vi "Teleop_debugging.vi"(10 "Match Info":T1={"Autonomous Elapsed Seconds"=0.0, "TeleOp Elapsed Seconds"=0.0, "Disabled Elapsed Seconds"=0.0, "Visited Autonomous"=FALSE, "Visited TeleOp"=FALSE, "Visited Disabled"=FALSE, "Autonomous Settings"={"Autonomous Style"=enum."Independent", "VI Refnum"=refnum}}, 11 "Call Context":T2) -> ()   [LabVIEW 2011]
doc: "This VI is called for each TeleOp packet received from the DS where the robot is not disabled. It is often used to read from the joysticks and update I/O or to update setpoints for timed control loops. It should complete and return within 20 milliseconds or it may miss DS packets."
uses:
  <vilib>/Rock Robotics/WPI/DriverStation/WPI_DriverStationDerivedRobotMode.ctl
  <vilib>/Rock Robotics/WPI/DriverStation/WPI_DriverStationMatch Info.ctl
  <vilib>/Rock Robotics/WPI/DriverStation/DriverStationLCD/WPI_DriverStationLCDLCDLine.ctl
  Robot Global Data.vi
  <vilib>/Rock Robotics/WPI/RobotDrive/WPI_RobotDriveMecanumDrive_Cartesian.vi
  <vilib>/addons/control/pid/NI_PID_pid.lvlib
panel:
  in  "ShooterAngle3":cluster{"time":dbl, "Arm Pos 1":dbl}[](array[cluster])=[{"time"=2.2540983606557377, "Arm Pos 1"=-0.5639931736228638}] {"Arm Pos 1" scale=1.0..-1.0 scale format="%#_4g"; "time" scale=0.0..5.0}
  in  "ShooterAngle2":cluster{"time":dbl, "Arm Pos 1":dbl}[](array[cluster])=[{"time"=2.2540983606557377, "Arm Pos 1"=-0.5639931736228638}] {"Arm Pos 1" scale=1.0..-1.0 scale format="%#_4g"; "time" scale=0.0..5.0}
  in  "ShooterAngle1":cluster{"time":dbl, "Arm Pos 1":dbl}[](array[cluster])=[{"time"=2.2540983606557377, "Arm Pos 1"=-0.5639931736228638}] {"Arm Pos 1" scale=1.0..-1.0 scale format="%#_4g"; "time" scale=0.0..5.0}
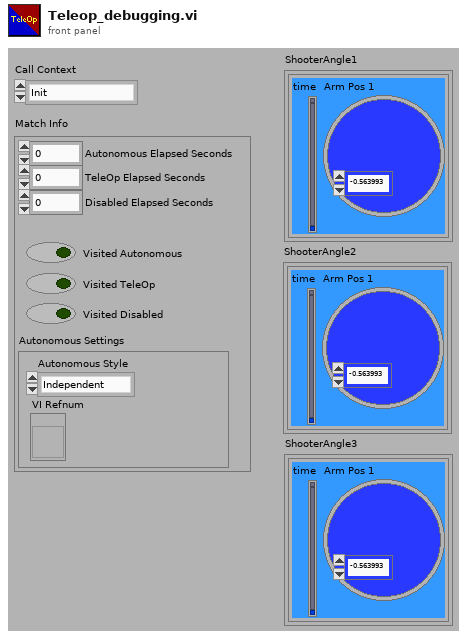
[diagram p1: front panel]
types:
  T1 = typedef "WPI_DriverStationMatch Info.ctl" = cluster{"Autonomous Elapsed Seconds":dbl, "TeleOp Elapsed Seconds":dbl, "Disabled Elapsed Seconds":dbl, "Visited Autonomous":bool, "Visited TeleOp":bool, "Visited Disabled":bool, "Autonomous Settings":cluster{"Autonomous Style":enum16{"Iterative", "Independent"}, "VI Refnum":refnum<vi>}}
  T2 = typedef "WPI_DriverStationDerivedRobotMode.ctl" = enum16{"Init", "Execute", "Stop"}
  T3 = typedef "WPI_DriverStationLCDLCDLine.ctl" = enum16{"Main - Line 1", "User - Line 2", "User - Line 3", "User - Line 4", "User - Line 5", "User - Line 6"}
  T4 = typedef "WPI_JoystickDevRef.ctl" = cluster{"Device":T5}
  T5 = typedef "WPI_JoystickDeviceEnum.ctl" = enum16{"USB 1", "USB 2", "USB 3", "USB 4", "Kinect 1", "Kinect 2"}
  T6 = typedef "WPI_MotorControlDeviceRef.ctl" = cluster{"DeviceStatus":errorcluster, "Type":enum16{"PWM", "CAN"}, "PWM":cluster{"Digital Module":T7, "PWM Channel":T8, "DeadBand":T9}, "CAN":cluster{"Device Number":u8, "Control Mode":T10, "Semaphore":T11, "Max Vout":dbl}, "Invert":bool, "TransformRef":T12, "InvTransformRef":T12}
  T7 = typedef "FPGA_TypedefDigitalModule.ctl" = enum16{"Digital Module 1", "Digital Module 2"}
  T8 = typedef "FPGA_DIOPWMChannel.ctl" = enum8{"PWM 1", "PWM 2", "PWM 3", "PWM 4", "PWM 5", "PWM 6", "PWM 7", "PWM 8", "PWM 9", "PWM 10", "Invalid"}
  T9 = typedef "WPI_PWMDeadband.ctl" = cluster{"Name":string, "maxPositivePwm":i32, "minPositivePwm":i32, "centerPwm":i32, "maxNegativePwm":i32, "minNegativePwm":i32, "angularRange":u16}
  T10 = typedef "WPI_CANJaguar_ControlMode.ctl" = enum8{"Percent VBus", "Current", "Speed", "Position", "Voltage"}
  T11 = typedef "Semaphore RefNum" = refnum<k1>
  T12 = typedef "WPI_PWMTransform_ConPane.ctl" = refnum<vi>
  T13 = cluster{"axis 1 (x)":dbl, "axis 2 (y)":dbl, "axis 3 (throttle)":dbl, "axis 4":dbl, "axis 5":dbl, "axis 6":dbl}
  T14 = typedef "WPI_JoystickButtonState.ctl" = cluster{"Button 1":bool, "Button 2":bool, "Button 3":bool, "Button 4":bool, "Button 5":bool, "Button 6":bool, "Button 7":bool, "Button 8":bool, "Button 9":bool, "Button 10":bool, "Button 11":bool, "Button 12":bool}
  T15 = typedef "WPI_ServoDeviceRef.ctl" = cluster{"DeviceStatus":errorcluster, "Digital Module":T7, "PWM Channel":T8, "DeadBand":T9}
  T16 = typedef "WPI_RobotDriveDevRef.ctl" = cluster{"DevStatus":errorcluster, "Motors[]":T6[], "Square Inputs":bool, "Max Output":dbl, "Isochronous":bool}
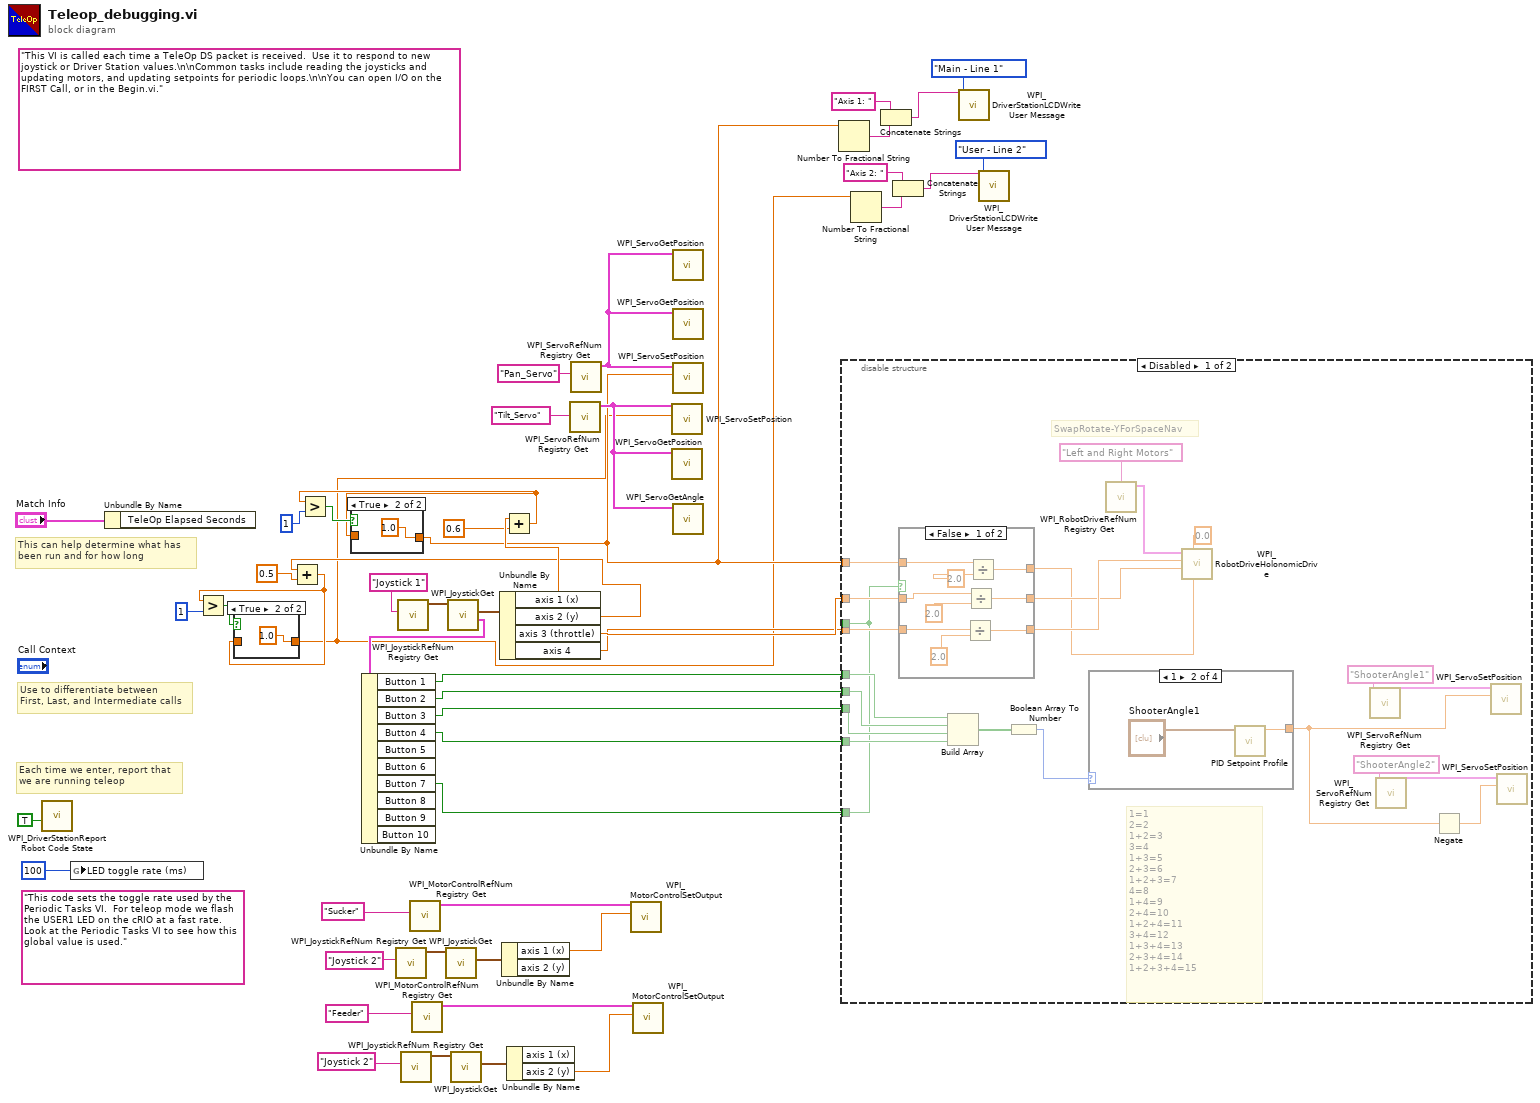
[diagram p0: block diagram]
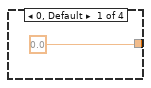
[diagram p4: hidden frame]
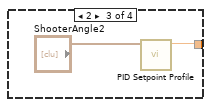
[diagram p5: hidden frame]
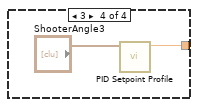
[diagram p6: hidden frame]
diagram:
  (unwired) "This code sets the toggle rate used by the Periodic Tasks VI.  For teleop mode we flash the USER1 LED on the cRIO at a fast rate.  Look at the Periodic Tasks VI to see how this global value is used."
  (unwired) "This VI is called each time a TeleOp DS packet is received.  Use it to respond to new joystick or Driver Station values.\n\nCommon tasks include reading the joysticks and updating motors, and updating setpoints for periodic loops.\n\nYou can open I/O on the FIRST Call, or in the Begin.vi."
  # "Each time we enter, report that\nwe are running teleop"
  # "Use to differentiate between\nFirst, Last, and Intermediate calls"
  # "This can help determine what has\nbeen run and for how long"
  n1 = call <vilib>:"WPI_DriverStationReport Robot Code State.vi"("TeleOp"=TRUE ("Autonomous")) -> ()  [unwired: 10 in, 1 out]
  n2 = global write "Robot Global Data.vi" "LED toggle rate (ms)"(u32 100 ("LED ms toggle rate")) -> ()
  n3 = Unbundle By Name("Match Info") -> ()  [unwired: 1 out]
  n4 = call <vilib>:"WPI_JoystickRefNum Registry Get.vi"("refnum name"="Joystick 2") -> ("JoystickDevRef"=w45:T4)  [unwired: 1 in, 9 out]
  n5 = call <vilib>:"WPI_JoystickRefNum Registry Get.vi"("refnum name"="Joystick 1") -> ("JoystickDevRef"=w33:T4)  [unwired: 1 in, 9 out]
  n6 = call <vilib>:"WPI_JoystickRefNum Registry Get.vi"("refnum name"="Joystick 2") -> ("JoystickDevRef"=w39:T4)  [unwired: 1 in, 9 out]
  n7 = call <vilib>:"WPI_MotorControlRefNum Registry Get.vi"("refnum name"="Sucker") -> ("MotorControlDevRef"=w44:T6)  [unwired: 9 in, 1 out]
  n8 = call <vilib>:"WPI_MotorControlRefNum Registry Get.vi"("refnum name"="Feeder") -> ("MotorControlDevRef"=w38:T6)  [unwired: 9 in, 1 out]
  n9 = call <vilib>:"WPI_JoystickGet.vi"("JoystickDevRef"=w45) -> ("Axes"=w47:T13)  [unwired: 1 in, 5 out]
  n10 = call <vilib>:"WPI_JoystickGet.vi"("JoystickDevRef"=w33) -> ("Buttons"=w32:T14, "Axes"=w35:T13)  [unwired: 1 in, 4 out]
  n11 = Unbundle By Name(w32) -> ("Button 1"=w29:bool, "Button 2"=w28:bool, "Button 3"=w27:bool, "Button 4"=w26:bool, "Button 7"=w25:bool)  [unwired: 5 out]
  n12 = call <vilib>:"WPI_JoystickGet.vi"("JoystickDevRef"=w39) -> ("Axes"=w41:T13)  [unwired: 1 in, 5 out]
  n13 = Unbundle By Name(w35) -> ("axis 1 (x)"=w12:dbl, "axis 2 (y)"=w6:dbl, "axis 3 (throttle)"=w31:dbl, "axis 4"=w30:dbl)
  n14 = Add(x=w6, y=0.5) -> (x+y=w2:dbl)
  n15 = Greater?(x=w2, y=1) -> (0:w3:bool)
  n16 = case shown="True" w3 {
    tunnel: w2 -> [w51 _]
    tunnel: [w51 1.0] -> w1
    frame False {
    }
    frame True {
    }
  }
  n17 = Unbundle By Name(w47) -> ("axis 1 (x)"=w42:dbl)  [unwired: 1 out]
  n18 = Add(x=w12, y=0.6) -> (x+y=w8:dbl)
  n19 = Greater?(x=w8, y=1) -> (0:w10:bool)
  n20 = case shown="True" w10 {
    tunnel: w8 -> [w53 _]
    tunnel: [w53 1.0] -> w7
    frame False {
    }
    frame True {
    }
  }
  n21 = Unbundle By Name(w41) -> ("axis 2 (y)"=w36:dbl)  [unwired: 1 out]
  n22 = call <vilib>:"WPI_ServoRefNum Registry Get.vi"("refnum name"="Tilt_Servo") -> ("ServoDeviceRef"=w23:T15)  [unwired: 9 in, 1 out]
  n23 = call <vilib>:"WPI_ServoRefNum Registry Get.vi"("refnum name"="Pan_Servo") -> ("ServoDeviceRef"=w21:T15)  [unwired: 9 in, 1 out]
  n24 = call <vilib>:"WPI_MotorControlSetOutput.vi"("Output"=w42, "MotorControlDevRef"=w44) -> ()  [unwired: 8 in, 2 out]
  n25 = call <vilib>:"WPI_MotorControlSetOutput.vi"("Output"=w36, "MotorControlDevRef"=w38) -> ()  [unwired: 8 in, 2 out]
  n26 = call <vilib>:"WPI_ServoSetPosition.vi"("Position"=w1, "ServoDeviceRef"=w23) -> ()  [unwired: 8 in, 2 out]
  n27 = call <vilib>:"WPI_ServoGetPosition.vi"("ServoDeviceRef"=w23) -> ()  [unwired: 8 in, 3 out]
  n28 = call <vilib>:"WPI_ServoGetPosition.vi"("ServoDeviceRef"=w21) -> ()  [unwired: 8 in, 3 out]
  n29 = call <vilib>:"WPI_ServoGetPosition.vi"("ServoDeviceRef"=w21) -> ()  [unwired: 8 in, 3 out]
  n30 = call <vilib>:"WPI_ServoSetPosition.vi"("Position"=w7, "ServoDeviceRef"=w21) -> ()  [unwired: 8 in, 2 out]
  n31 = call <vilib>:"WPI_ServoGetAngle.vi"("ServoDeviceRef"=w23) -> ()  [unwired: 7 in, 3 out]
  n32 = Number To Fractional String(number=w7) -> (F-format string=w18:string)  [unwired: 3 in]
  n33 = disable-structure shown="Disabled" {
    disable-tunnel: w31 -> [w76 _]
    disable-tunnel: w30 -> [w75 _]
    disable-tunnel: w29 -> [w63 _]
    disable-tunnel: w28 -> [w62 _]
    disable-tunnel: w27 -> [w61 _]
    disable-tunnel: w26 -> [w60 _]
    disable-tunnel: w7 -> [w56 _]
    disable-tunnel: [w55 _] -> _
    disable-tunnel: w25 -> [w55 _]
    frame Disabled {
      # "1=1\n2=2\n1+2=3\n3=4\n1+3=5\n2+3=6\n1+2+3=7\n4=8\n1+4=9\n2+4=10\n1+2+4=11\n3+4=12\n1+3+4=13\n2+3+4=14\n1+2+3+4=15"
      # "SwapRotate-YForSpaceNav"
      n34 = case shown="False" w55 {
        tunnel: w75 -> [w87 w95]
        tunnel: [w86 w95] -> w71
        tunnel: w76 -> [w85 w94]
        tunnel: [w90 w94] -> w70
        tunnel: w56 -> [w89 w93]
        tunnel: [w84 w93] -> w69
        frame False {
          n35 = Divide(x=w87, y=2.0) -> (x/y=w86:dbl)
          n36 = Divide(x=w85, y=2.0) -> (x/y=w90:dbl)
          n37 = Divide(x=w89, y=2.0) -> (x/y=w84:dbl)
        }
        frame True {
        }
      }
      n38 = Build Array(w63, w62, w61, w60) -> (w59:bool[])
      n39 = Boolean Array To Number(Boolean array=w59) -> (number=w58:u32)
      n40 = case shown="1" w58 {
        tunnel: [0.0 w78 w80 w82] -> w57
        frame 0, Default {
        }
        frame 1 {
          n41 = call <vilib>:"PID Setpoint Profile.vi"("setpoint profile"="ShooterAngle1") -> ("setpoint"=w78:dbl)  [unwired: 2 in, 6 out]
        }
        frame 2 {
          n42 = call <vilib>:"PID Setpoint Profile.vi"("setpoint profile"="ShooterAngle2") -> ("setpoint"=w80:dbl)  [unwired: 2 in, 6 out]
        }
        frame 3 {
          n43 = call <vilib>:"PID Setpoint Profile.vi"("setpoint profile"="ShooterAngle3") -> ("setpoint"=w82:dbl)  [unwired: 2 in, 6 out]
        }
      }
      n44 = call <vilib>:"WPI_RobotDriveRefNum Registry Get.vi"("refnum name"="Left and Right Motors") -> ("RobotDriveDevRef"=w73:T16)  [unwired: 1 in, 9 out]
      n45 = call-poly <vilib>:"WPI_RobotDriveHolonomicDrive.vi"("Rotation"=w69, "Gyro Angle"=0.0, "Y"=w70, "X"=w71, "RobotDriveDevRef"=w73) -> ()  [unwired: 1 in, 6 out]
      n46 = call <vilib>:"WPI_ServoRefNum Registry Get.vi"("refnum name"="ShooterAngle1") -> ("ServoDeviceRef"=w67:T15)  [unwired: 1 in, 9 out]
      n47 = call <vilib>:"WPI_ServoRefNum Registry Get.vi"("refnum name"="ShooterAngle2") -> ("ServoDeviceRef"=w65:T15)  [unwired: 1 in, 9 out]
      n48 = Negate(x=w57) -> (-x=w64:dbl)
      n49 = call <vilib>:"WPI_ServoSetPosition.vi"("Position"=w57, "ServoDeviceRef"=w67) -> ()  [unwired: 1 in, 9 out]
      n50 = call <vilib>:"WPI_ServoSetPosition.vi"("Position"=w64, "ServoDeviceRef"=w65) -> ()  [unwired: 1 in, 9 out]
    }
    frame Enabled {
    }
  }
  n51 = Number To Fractional String(number=w1) -> (F-format string=w16:string)  [unwired: 3 in]
  n52 = Concatenate Strings("Axis 1: ", w18) -> (w15:string)
  n53 = Concatenate Strings("Axis 2: ", w16) -> (w13:string)
  n54 = call <vilib>:"WPI_DriverStationLCDWrite User Message.vi"("line text"=w15, "line"=WPI_DriverStationLCDLCDLine."Main - Line 1") -> ()  [unwired: 13 in, 1 out]
  n55 = call <vilib>:"WPI_DriverStationLCDWrite User Message.vi"("line text"=w13, "line"=WPI_DriverStationLCDLCDLine."User - Line 2") -> ()  [unwired: 13 in, 1 out]
